vi "Multiple Migration mockup UI.vi"() -> ()   [LabVIEW 2021]
uses:
  <vilib>/Utility/miscctls.llb/LVRowAndColumnTypeDef.ctl
panel:
  in  "Tab Control":T1(tab)
  in  "Select Measurement":path
  out "Warning":bool=TRUE caption="Warning:\nProject Location cannot be empty/invalid"
  in  "Next 1":bool
  in  "Select Project":path
  in  "Select all":bool
  in  "Back 1":bool
  in  "Next 2":bool
  in  "Select Measurements":string(tree)
  out "Selection warning":string="Atleast one measurement should be selected"
  in  "Start Migration":bool
  in  "Back 2":bool
  in  "List of Selected Measurements":i32(listbox)
  in  "Measurement Count":i32(slide)=6 caption="Migrating 3 of 3 Measurements" scale=0.0..10.0
  in  "Progress":i32(slide)=9 caption="Editing Measurement UI" scale=0.0..10.0
  in  "Error Log":bool
  in  "Review":bool
  in  "Migration Status":i32(listbox)
  in  "Back to Status":bool
  in  "Select Plug-in":string(combo) caption="Select Measurement plug-in to review"
  in  "Start Next":bool
  out "Launch Type Spec":string
  out "Launch Logic":string
  out "Launch UI":string
  # ".lvproj"
  # "* Project in which the measurement plug-in will be created"
  # "* Select a measurement vi or a folder containing measurements"
  # "Select the measurements to migrate"
  # "* Rename the Plug-in if required"
  # "Review the Measurement:\n1. Review the Measurement UI. Click here to launch.\n2. Review the Measurement Logic VI. Click here to launch.\n3. Review the Type Specialization VI. Click here to launch."
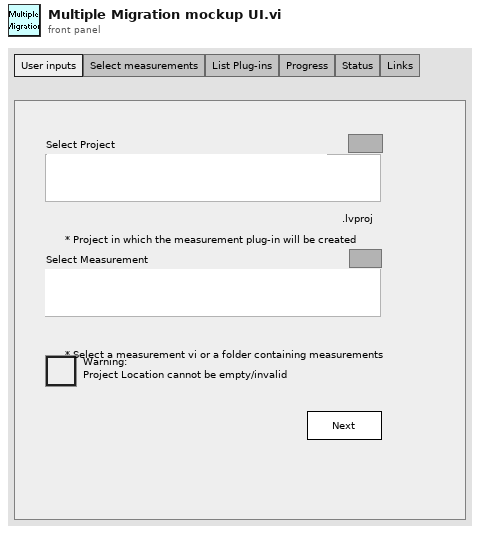
[diagram p1: front panel]
types:
  T1 = enum32{"User inputs", "Select measurements", "List Plug-ins", "Progress", "Status", "Links"}
  T2 = typedef "LVRowAndColumnTypeDef.ctl" = cluster{"Row":i32, "Column":i32}
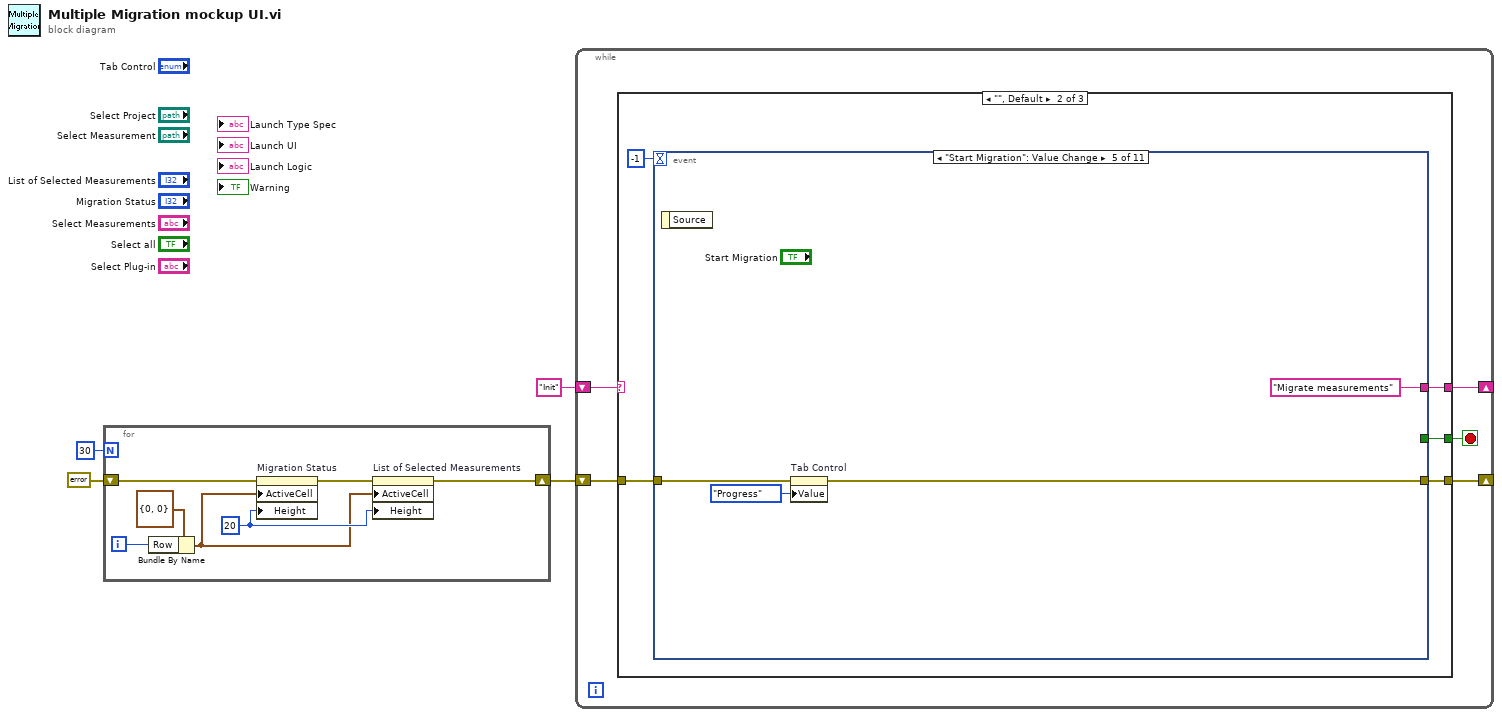
[diagram p0: block diagram]
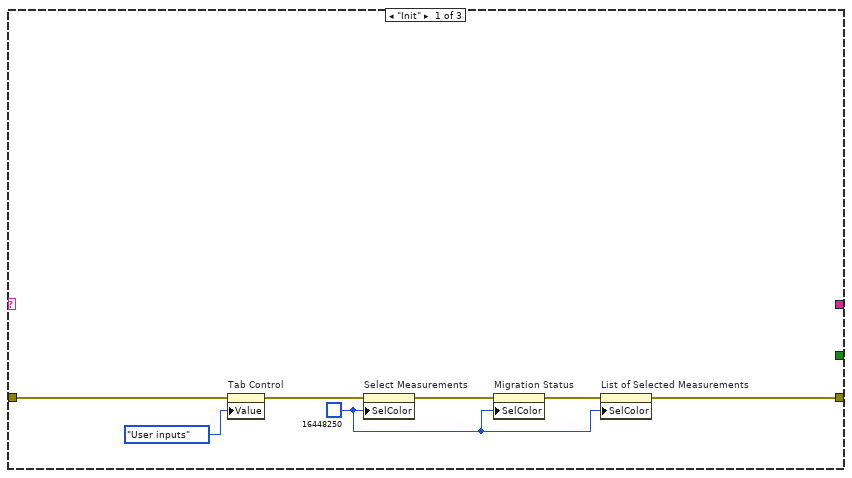
[diagram p2: hidden frame]
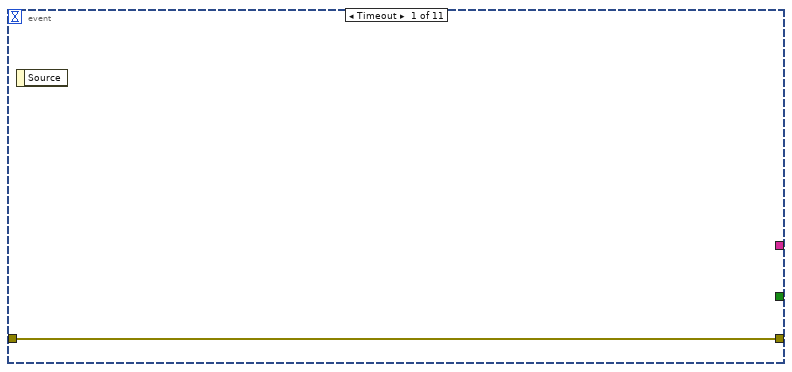
[diagram p3: hidden frame]
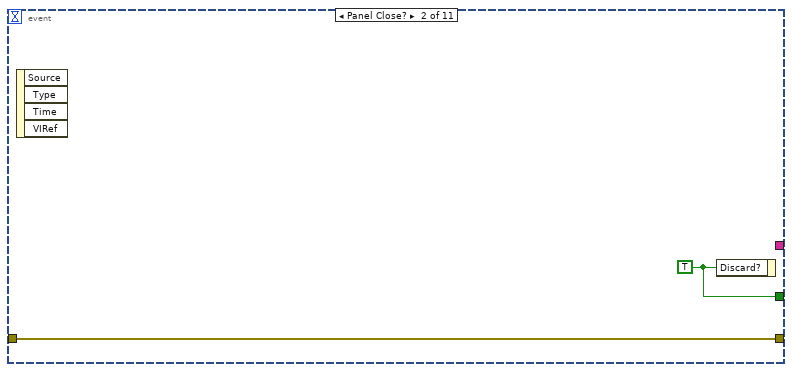
[diagram p4: hidden frame]
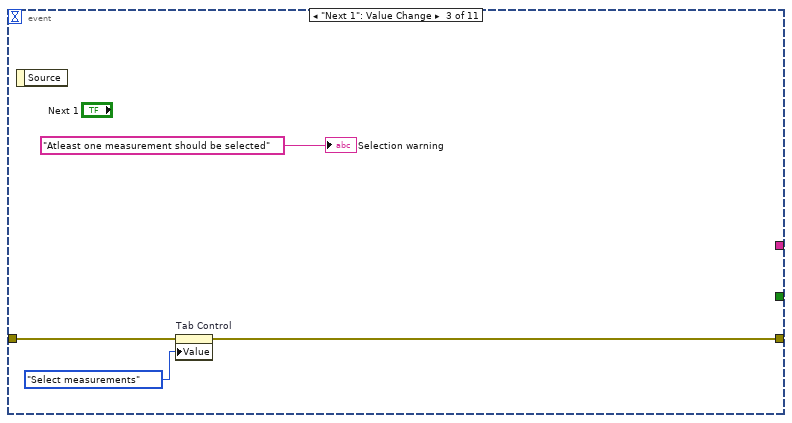
[diagram p5: hidden frame]
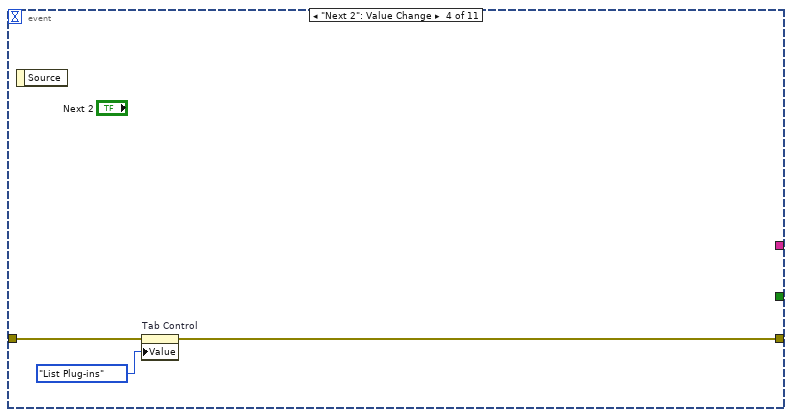
[diagram p6: hidden frame]
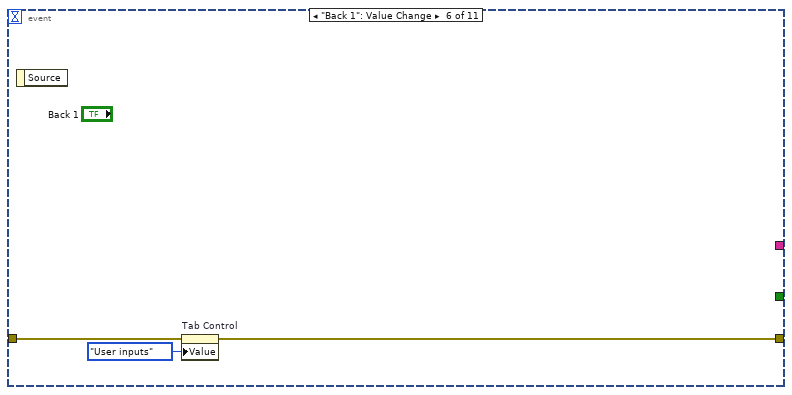
[diagram p7: hidden frame]
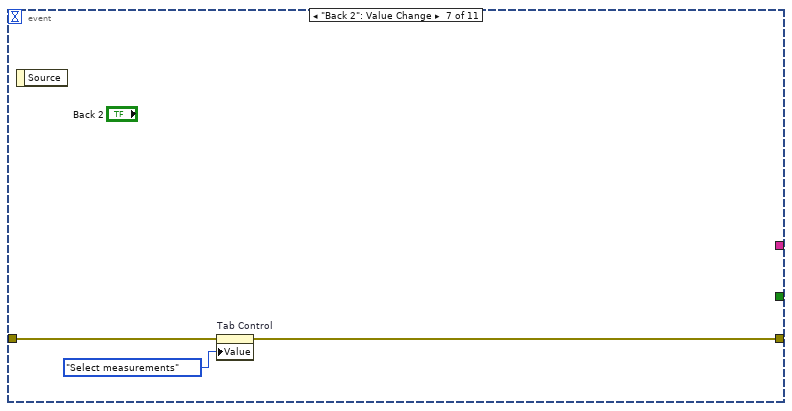
[diagram p8: hidden frame]
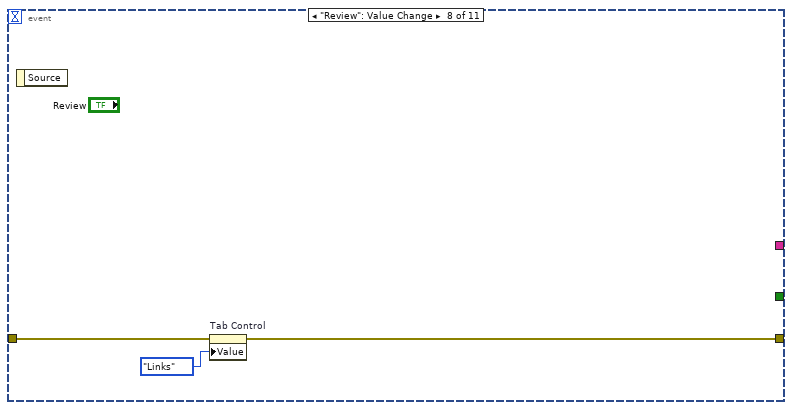
[diagram p9: hidden frame]
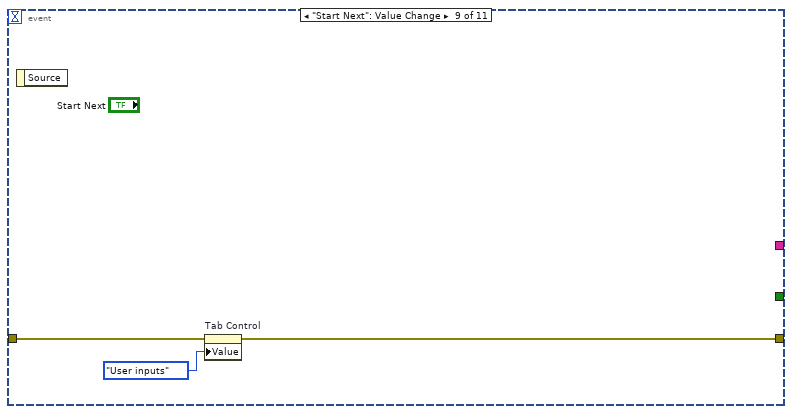
[diagram p10: hidden frame]
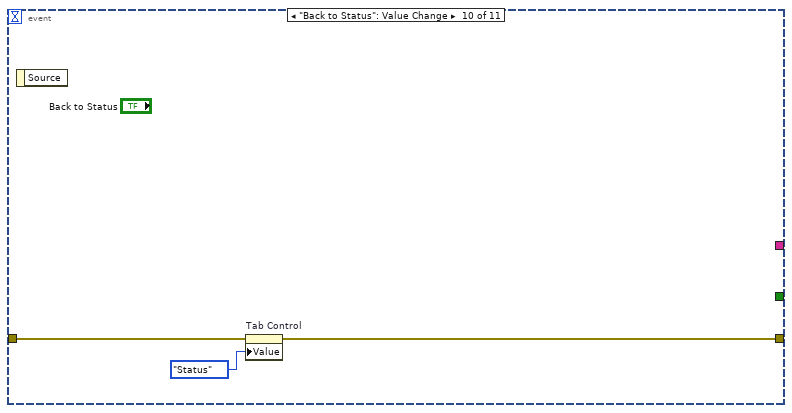
[diagram p11: hidden frame]
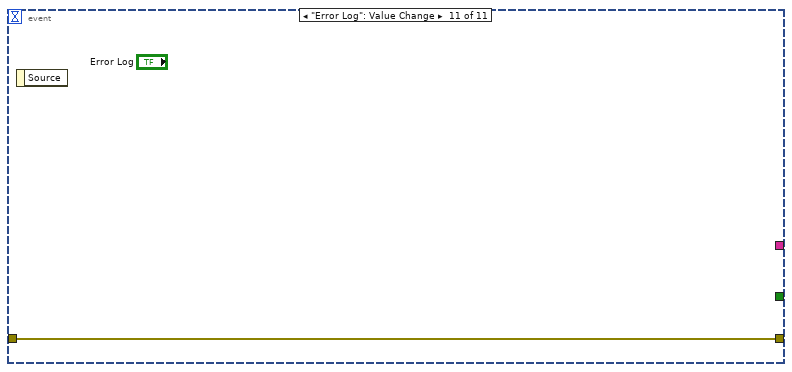
[diagram p12: hidden frame]
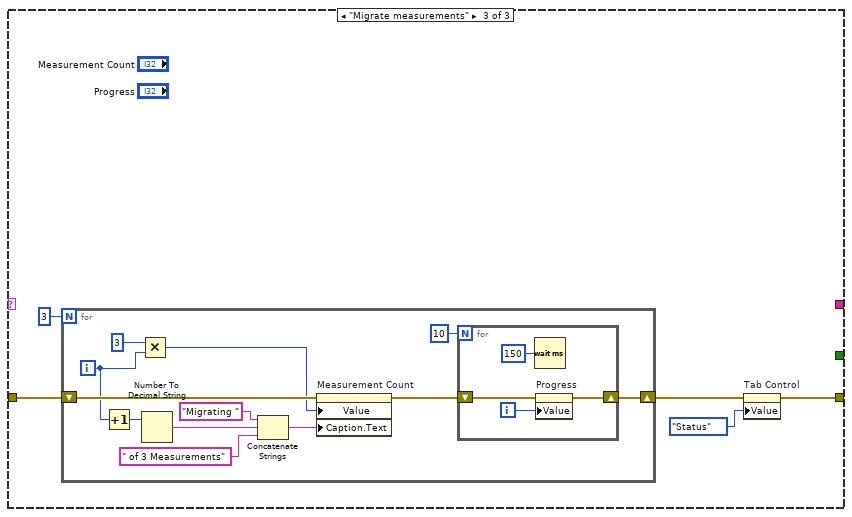
[diagram p13: hidden frame]
diagram:
  n1 = for {
    N: 30 -> [_]
    shift-right: [w9] -> w1
    shift-left: errorcluster {"status"=FALSE, "code"=0, "source"=""} ("error in (no error)") -> [w6]
    i -> [w10]
    w8 = u32 20 ("Active Cell:Cell Size:Height")
    n2 = Bundle By Name(cluster=T2 {"Row"=0, "Column"=0} ("Active Cell:Active Cell"), "Row"=w10) -> (w7:T2)
    n3 = property on="Migration Status" class="MCListbox (strict)"(error in=w6, "ActiveCell"=w7, "Height"=w8) -> (error out=w5:errorcluster)  [unwired: 1 in, 1 out]
    n4 = property on="List of Selected Measurements" class="MCListbox (strict)"(error in=w5, "ActiveCell"=w7, "Height"=w8) -> (error out=w9:errorcluster)  [unwired: 1 in, 1 out]
  }
  n5 = while {
    shift-right: [w14] -> _
    shift-left: w1 -> [w15]
    shift-right: [w12] -> _
    shift-left: "Init" -> [w13]
    stop <- w16 stop-if-true
    n6 = case shown="\"\", Default" w13 {
      tunnel: [_ w27 _] -> w16
      tunnel: w15 -> [w23 w26 w63]
      tunnel: [w18 w25 w61] -> w14
      tunnel: [_ w24 _] -> w12
      frame "Init" {
        w17 = u32 16448250 ("Selection Color")
        n7 = property on="Tab Control" class="TabCtl (strict)"(error in=w23, "Value"=T1."User inputs" ("Tab Control")) -> (error out=w19:errorcluster)  [unwired: 1 in, 1 out]
        n8 = property on="Select Measurements" class="Tree (strict)"(error in=w19, "SelColor"=w17) -> (error out=w21:errorcluster)  [unwired: 1 in, 1 out]
        n9 = property on="Migration Status" class="MCListbox (strict)"(error in=w21, "SelColor"=w17) -> (error out=w20:errorcluster)  [unwired: 1 in, 1 out]
        n10 = property on="List of Selected Measurements" class="MCListbox (strict)"(error in=w20, "SelColor"=w17) -> (error out=w18:errorcluster)  [unwired: 1 in, 1 out]
      }
      frame "", Default {
        n11 = event shown="[4] \"Start Migration\": Value Change" {
          selector: _ -> [_ _ _ _ _ _ _ _ _ _ _]
          dyn-events: _ -> [_ _ _ _ _ _ _ _ _ _ _]
          timeout: -1 -> [_ _ _ _ _ _ _ _ _ _ _]
          tunnel: [_ w31 _ _ _ _ _ _ _ _ _] -> w27
          tunnel: w26 -> [w29 w30 w35 w38 w42 w45 w48 w51 w54 w57 w58]
          tunnel: [w29 w30 w33 w36 w41 w44 w47 w50 w53 w56 w58] -> w25
          tunnel: [_ _ _ _ "Migrate measurements" _ _ _ _ _ _] -> w24
          event Timeout {
            n12 = event-data() -> ()  [unwired: 1 in, 1 out]
          }
          event Panel Close? {
            w31 = TRUE ("Discard?")
            n13 = event-data() -> ()  [unwired: 1 in, 4 out]
            n14 = event-data("Discard?"=w31) -> ()  [unwired: 1 in, 1 out]
          }
          event "Next 1": Value Change {
            n15 = event-data() -> ()  [unwired: 1 in, 1 out]
            n16 = property on="Tab Control" class="TabCtl (strict)"(error in=w35, "Value"=T1."Select measurements" ("Tab Control")) -> (error out=w33:errorcluster)  [unwired: 1 in, 1 out]
            "Selection warning" <- "Atleast one measurement should be selected" ("Selection warning")
          }
          event "Next 2": Value Change {
            n17 = event-data() -> ()  [unwired: 1 in, 1 out]
            n18 = property on="Tab Control" class="TabCtl (strict)"(error in=w38, "Value"=T1."List Plug-ins" ("Tab Control")) -> (error out=w36:errorcluster)  [unwired: 1 in, 1 out]
          }
          event "Start Migration": Value Change {
            n19 = event-data() -> ()  [unwired: 1 in, 1 out]
            n20 = property on="Tab Control" class="TabCtl (strict)"(error in=w42, "Value"=T1."Progress" ("Tab Control")) -> (error out=w41:errorcluster)  [unwired: 1 in, 1 out]
          }
          event "Back 1": Value Change {
            n21 = event-data() -> ()  [unwired: 1 in, 1 out]
            n22 = property on="Tab Control" class="TabCtl (strict)"(error in=w45, "Value"=T1."User inputs" ("Tab Control")) -> (error out=w44:errorcluster)  [unwired: 1 in, 1 out]
          }
          event "Back 2": Value Change {
            n23 = event-data() -> ()  [unwired: 1 in, 1 out]
            n24 = property on="Tab Control" class="TabCtl (strict)"(error in=w48, "Value"=T1."Select measurements" ("Tab Control")) -> (error out=w47:errorcluster)  [unwired: 1 in, 1 out]
          }
          event "Review": Value Change {
            n25 = event-data() -> ()  [unwired: 1 in, 1 out]
            n26 = property on="Tab Control" class="TabCtl (strict)"(error in=w51, "Value"=T1."Links" ("Tab Control")) -> (error out=w50:errorcluster)  [unwired: 1 in, 1 out]
          }
          event "Start Next": Value Change {
            n27 = event-data() -> ()  [unwired: 1 in, 1 out]
            n28 = property on="Tab Control" class="TabCtl (strict)"(error in=w54, "Value"=T1."User inputs" ("Tab Control")) -> (error out=w53:errorcluster)  [unwired: 1 in, 1 out]
          }
          event "Back to Status": Value Change {
            n29 = event-data() -> ()  [unwired: 1 in, 1 out]
            n30 = property on="Tab Control" class="TabCtl (strict)"(error in=w57, "Value"=T1."Status" ("Tab Control")) -> (error out=w56:errorcluster)  [unwired: 1 in, 1 out]
          }
          event "Error Log": Value Change {
            n31 = event-data() -> ()  [unwired: 1 in, 1 out]
          }
        }
      }
      frame "Migrate measurements" {
        n32 = for {
          N: 3 -> [_]
          shift-right: [w75] -> w62
          shift-left: w63 -> [w72]
          i -> [w64]
          n33 = Increment(x=w64) -> (x+1=w65:i32)
          n34 = Multiply(x=3 ("y"), y=w64) -> (x*y=w70:i32)
          n35 = Number To Decimal String(number=w65) -> (decimal integer string=w67:string)  [unwired: 1 in]
          n36 = Concatenate Strings("Migrating " ("string"), w67, " of 3 Measurements" ("string")) -> (w68:string)
          n37 = property on="Measurement Count" class="Slide (strict)"(error in=w72, "Value"=w70, "Caption.Text"=w68) -> (error out=w71:errorcluster)  [unwired: 1 in, 1 out]
          n38 = for {
            N: 10 -> [_]
            shift-right: [w77] -> w75
            shift-left: w71 -> [w78]
            i -> [w76]
            n39 = Wait (ms)(milliseconds to wait=u32 150) -> ()  [unwired: 1 out]
            n40 = property on="Progress" class="Slide (strict)"(error in=w78, "Value"=w76) -> (error out=w77:errorcluster)  [unwired: 1 in, 1 out]
          }
        }
        n41 = property on="Tab Control" class="TabCtl (strict)"(error in=w62, "Value"=T1."Status" ("Tab Control")) -> (error out=w61:errorcluster)  [unwired: 1 in, 1 out]
      }
    }
  }
